vi "mn-430 control.vi"() -> ()   [LabVIEW 2011]
panel:
  out "connection ID out":refnum<k5>
  in  "stop":bool
  in  "Send":bool
  out "Init Response":string
  in  "Query":bool
  out "Response":string
  out "error out 2":errorcluster
  in  "error in (no error)":errorcluster
  in  "IP Address":string
  in  "Command":string
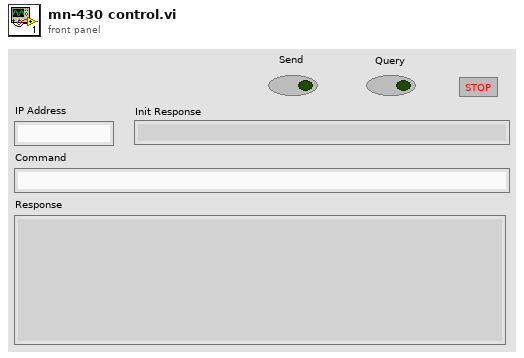
[diagram p1: front panel]
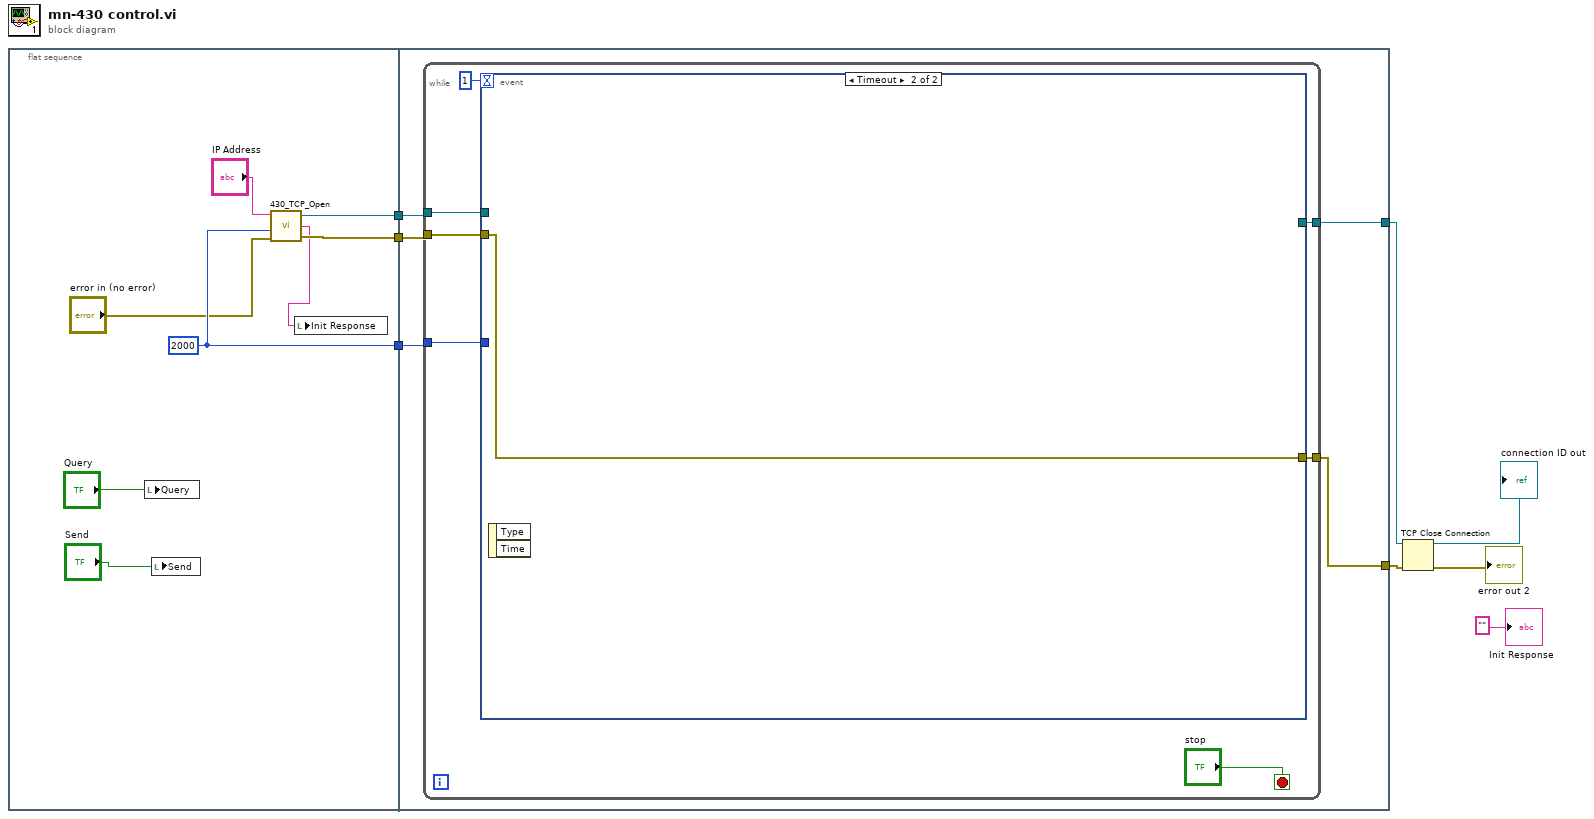
[diagram p0: block diagram]
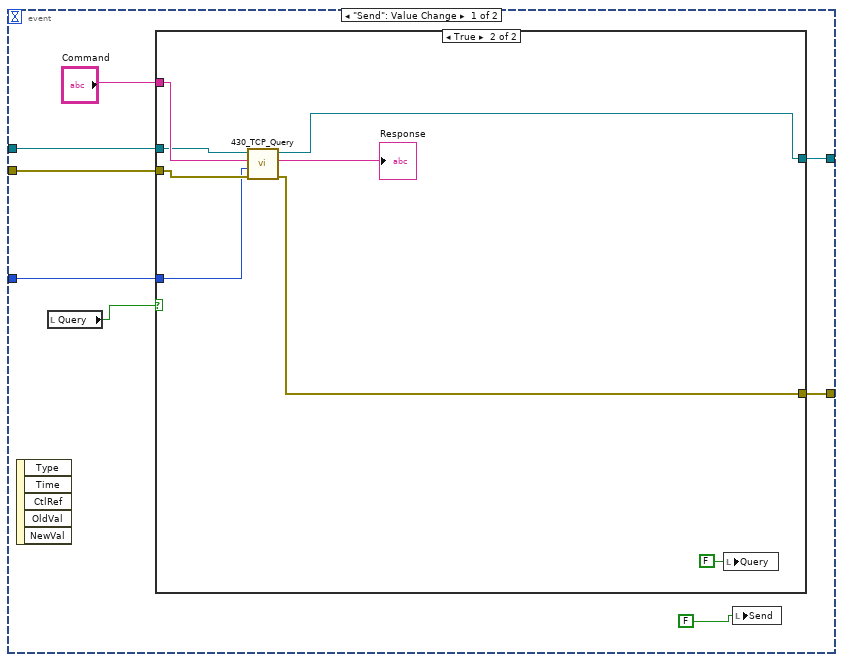
[diagram p2: hidden frame]
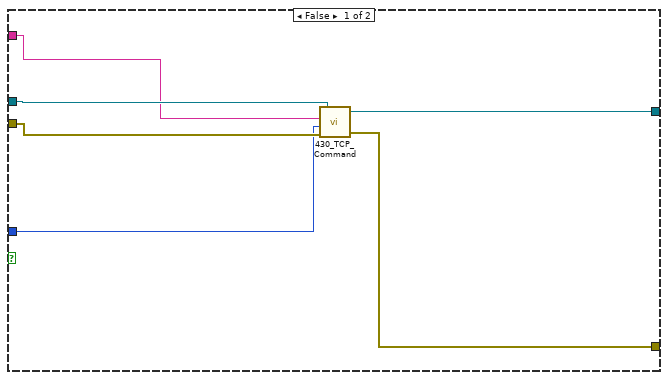
[diagram p3: hidden frame]
diagram:
  n1 = flat-sequence {
    tunnel: [w16] -> w8
    tunnel: [w15] -> w7
    tunnel: [w13] -> w6
    tunnel: w8 -> [w20]
    tunnel: w7 -> [w21]
    tunnel: w6 -> [w19]
    tunnel: [w18] -> w5
    tunnel: [w17] -> w3
    frame #0 {
      w13 = 2000 ("Timeout")
      n2 = local write "Query"("Query") -> ()
      n3 = local write "Send"("Send") -> ()
      n4 = call "430_TCP_Open.vi"("IP Address"="IP Address", "timeout ms (2000)"=w13, "error in (no error)"="error in (no error)") -> ("connection ID"=w15:refnum<k5>, "Init Response"=w9:string, "error out"=w16:errorcluster)  [unwired: 3 in]
      n5 = local write "Init Response"(w9) -> ()
    }
    frame #1 {
      n6 = while {
        tunnel: w20 -> [w28]
        tunnel: w21 -> [w27]
        tunnel: w19 -> [w26]
        tunnel: [w25] -> w18
        tunnel: [w22] -> w17
        stop <- "stop" stop-if-true
        n7 = event shown="[1] Timeout" {
          selector: _ -> [_ _]
          dyn-events: _ -> [_ _]
          timeout: 1 -> [_ _]
          tunnel: w28 -> [w36 w51]
          tunnel: w27 -> [w35 _]
          tunnel: w26 -> [w34 _]
          tunnel: [w33 w51] -> w25
          tunnel: [w29 _] -> w22
          event "Send": Value Change {
            n8 = event-data() -> ()  [unwired: 1 in, 5 out]
            n9 = local read "Query"() -> (w31:bool)
            n10 = case shown="True" w31 {
              tunnel: w36 -> [w41 w49]
              tunnel: w35 -> [w42 w43]
              tunnel: w34 -> [w40 w48]
              tunnel: [w39 w47] -> w33
              tunnel: "Command" -> [w38 w50]
              tunnel: [w37 w46] -> w29
              frame False {
                n11 = call "430_TCP_Command.vi"("error in (no error)"=w41, "Timeout"=w40, "Command"=w38, "connection ID"=w42) -> ("error out"=w39:errorcluster, "connection ID out"=w37:refnum<k5>)  [unwired: 1 out]
              }
              frame True {
                n12 = call "430_TCP_Query.vi"("error in (no error)"=w49, "Timeout"=w48, "Command"=w50, "connection ID"=w43) -> ("error out"=w47:errorcluster, "Response"=→"Response":string, "connection ID out"=w46:refnum<k5>)  [unwired: 3 in, 2 out]
                n13 = local write "Query"(FALSE ("Query")) -> ()
              }
            }
            n14 = local write "Send"(FALSE ("Send")) -> ()
          }
          event Timeout {
            n15 = event-data() -> ()  [unwired: 1 in, 2 out]
          }
        }
      }
    }
  }
  n16 = TCP Close Connection(connection ID=w3, error in (no error)=w5) -> (connection ID out=→"connection ID out":refnum<k5>, error out=→"error out 2":errorcluster)  [unwired: 1 in]
  "Init Response" <- "" ("Init Response")
